vi "Utility Recall Setting Mode.vi"(0 "VISA resource name":refnum<visa-resource-name>, 7 "Recall State (0:Setting 1)":T1(ring), 11 "error in (no error)":errorcluster) -> (4 "VISA resource name out":refnum<visa-resource-name>, 15 "error out":errorcluster)   [LabVIEW 2010, in "Stanford Research PS300 Series.lvlib"]
doc: "This VI recalls stored configuration setting from the instrument memory.If the stored setting is corrupted, an error is returned."
uses:
  <instrlib>/Stanford Research PS300 Series/Stanford Research PS300 Series.lvlib
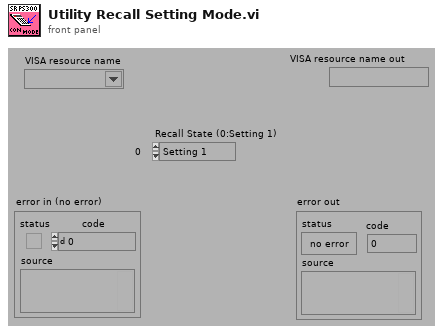
[diagram p1: front panel]
types:
  T1 = enum16{"Setting 1", "Setting 2", "Setting 3", "Setting 4", "Setting 5", "Setting 6", "Setting 7", "Setting 8", "Setting 9"}
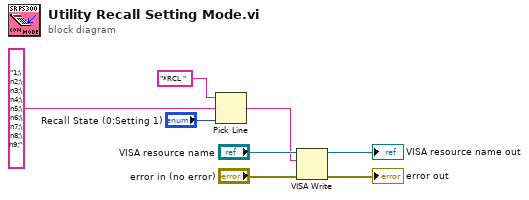
[diagram p0: block diagram]
diagram:
  n1 = Pick Line(string ("")="*RCL ", multi-line string="1;\n2;\n3;\n4;\n5;\n6;\n7;\n8;\n9;", line index="Recall State (0:Setting 1)") -> (output string=w1:string)
  n2 = VISA Write(VISA resource name="VISA resource name", write buffer=w1, error in (no error)="error in (no error)") -> (VISA resource name out=→"VISA resource name out":refnum<visa-resource-name>, error out=→"error out":errorcluster)  [unwired: 1 out]
